vi "Run Service.vi"   [LabVIEW 2020, in "Keysight 34401A DMM Measurement.lvlib"]
uses:
  Keysight 34401A DMM Measurement.lvlib
  Advanced/MeasurementPlugin.lvclass
  C:/Program Files/National Instruments/LabVIEW 2020/vi.lib/MeasurementLink/MeasurementLink Measurement Server/Classes/MeasurementPluginService/MeasurementPluginService.lvclass
  <vilib>/MeasurementLink/MeasurementLink Measurement Server/MeasurementLink Measurement Server.lvlib
  D:/dev/measurementlink-labview/Source/Example Measurements/Keysight 34401A DMM Measurement/Keysight 34401A DMM Measurement/Advanced/MeasurementPlugin.lvclass
panel:
  # "Run this VI to start the measurement service.  A window will appear that provides basic information about the running service.\n\nUse the stop button on the window that appears to stop the measurement service."
types:
  T1 = enum32{"Invalid", "Standard", "Closed", "Hidden", "Minimized", "Maximized"}
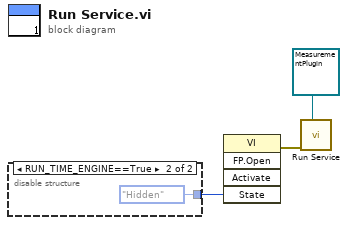
[diagram p0: block diagram]
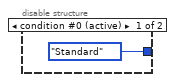
[diagram p2: hidden frame]
diagram:
  n1 = disable-structure shown="RUN_TIME_ENGINE==True" {
    disable-tunnel: [T1."Standard" ("State") T1."Hidden" ("State")] -> w3
    frame condition #0 (active) {
    }
    frame condition #1 {
    }
  }
  n2 = invoke class="VI" method="FP.Open"("State"=w3) -> (error out=w1:errorcluster)  [unwired: 4 in, 4 out]
  n3 = call <vilib>:"Run Service.vi"("Measurement"=refnum<class "MeasurementPlugin.lvclass"> refnum ("MeasurementLink Measurement Template.lvlib:Measurement Customizations.lvclass"), "error in (no error)"=w1) -> ()  [unwired: 10 in]
